vi "2b.vi"() -> ()   [LabVIEW 2015]
panel:
  in  "Cluster":cluster{"Array":dbl[][]}
  out "Waveform Graph":dbl[][](graph)
  in  "# of samples/channel":i32=1000
  in  "Sampling rate":dbl=10000.0
  in  "physical channels":tag="Dev1/ai0:2"
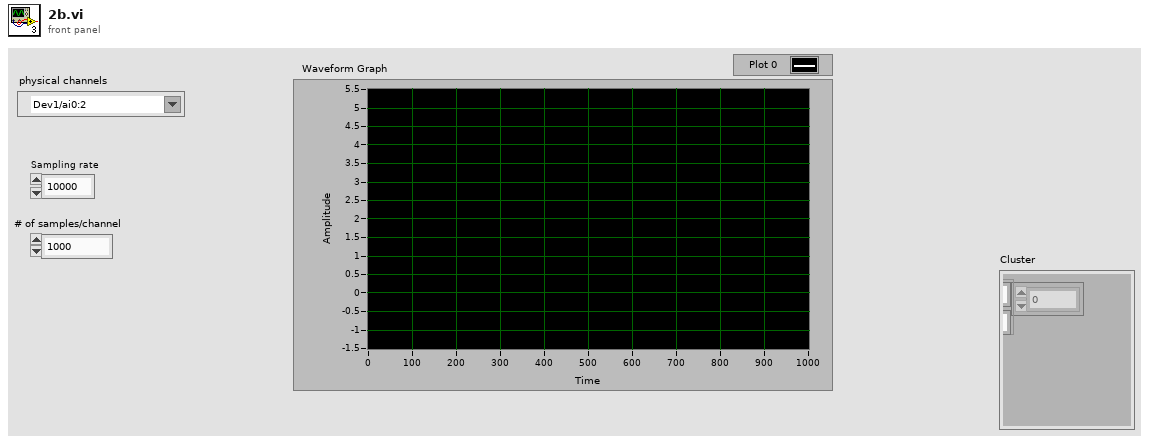
[diagram p1: front panel]
types:
  T1 = enum16{"open", "replace", "create", "open or create", "replace or create", "replace or create with confirmation"}
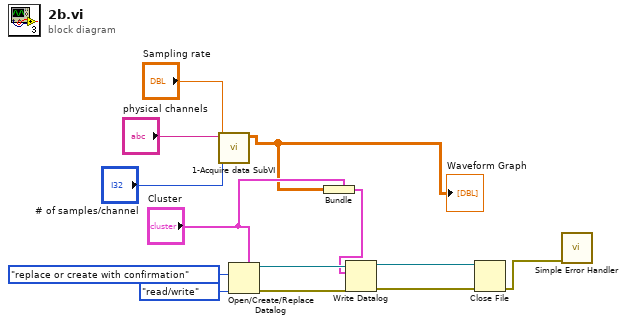
[diagram p0: block diagram]
diagram:
  n1 = call "1-Acquire data SubVI.vi"("# of samples/channel"="# of samples/channel", "Sampling rate"="Sampling rate", "physical channels"="physical channels") -> ("data"=w2:dbl[][])  [unwired: 8 in]
  "Waveform Graph" <- w2
  n2 = Open/Create/Replace Datalog(5:"Cluster", 9:enum16{"read/write", "read-only", "write-only"}."read/write" ("access (0:read/write)"), 10:T1."replace or create with confirmation" ("operation (0:open)")) -> (0:w10:errorcluster, 3:w5:refnum<k1>)  [unwired: 3 in, 1 out]
  n3 = Bundle(cluster="Cluster", "Array"=w2) -> (w3:cluster{"Array":dbl[][]})
  n4 = Write Datalog(4:w10, 6:w3, 7:w5) -> (0:w9:errorcluster, 3:w8:refnum<k1>)
  n5 = Close File(refnum=w8, error in=w9) -> (error out=w1:errorcluster)  [unwired: 1 out]
  n6 = call <vilib>:"Simple Error Handler.vi"("error in (no error)"=w1) -> ()  [unwired: 4 in, 5 out]
